vi "Script IO Nodes.vi"(5 "Device Info":T1, 6 "Number of SPI Buses":i32, 7 "Curent Bus Path":path, 8 "error in (no error)":errorcluster, 9 "Device Channels":i32[](array[numeric]), 11 "LabVIEW Project to Script":path) -> (0 "error out":errorcluster, 3 "New Node Paths":path[](array[path]))   [LabVIEW 2014, in "Initialization and IO Node Scripting.lvlib"]
uses:
  Initialization and IO Node Scripting.lvlib
  State Machine/Controls/Bus Information.ctl
  State Machine/Controls/Device Information.ctl
  State Machine/Controls/Pin Information.ctl
  State Machine/Controls/Values for Naming.ctl
panel:
  in  "New Virtual Folder":refnum<vi>
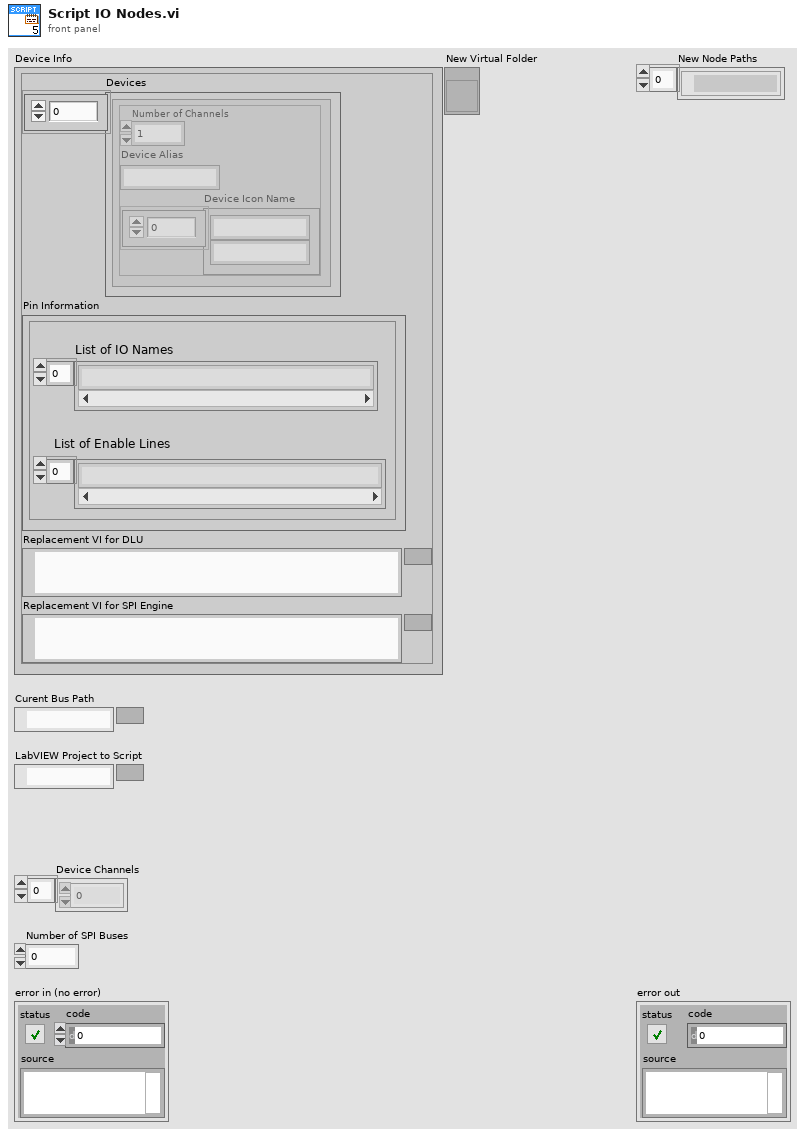
[diagram p1: front panel]
types:
  T1 = typedef "Initialization and IO Node Scripting.lvlib/Bus Information.ctl" = cluster{"Devices":T2[], "Pin Information":T3, "Replacement VI for DLU":path, "Replacement VI for SPI Engine":path}
  T2 = typedef "Device Information.ctl" = cluster{"Number of Channels":i32, "Device Alias":string, "Device Icon Name":string[]}
  T3 = typedef "Pin Information.ctl" = cluster{"List of IO Names":string[], "List of Enable Lines":string[]}
  T4 = typedef "Initialization and IO Node Scripting.lvlib/Values for Naming.ctl" = cluster{"Bus Number":i32, "Device Number":i32, "Channel Number":i32}
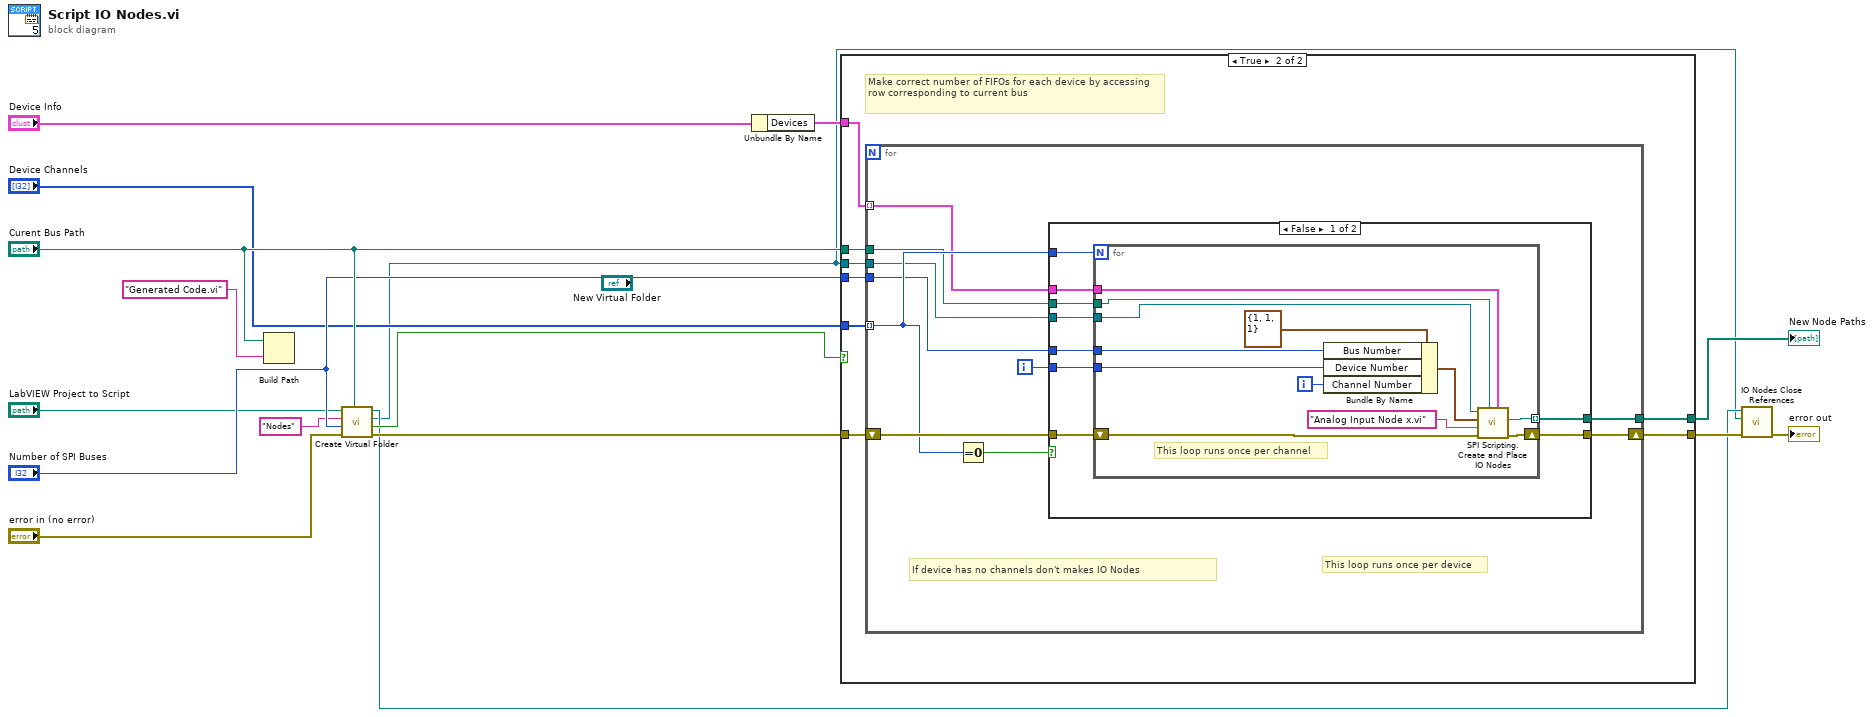
[diagram p0: block diagram]
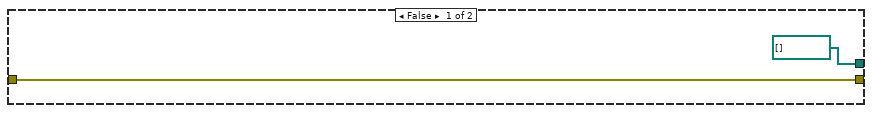
[diagram p2: hidden frame]
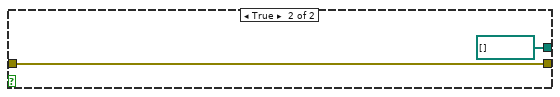
[diagram p3: hidden frame]
diagram:
  n1 = Build Path(base path="Curent Bus Path", name or relative path="Generated Code.vi") -> ()  [unwired: 1 out]
  n2 = call "Create Virtual Folder.vi"("Curent Bus Path"="Curent Bus Path", "error in"="error in (no error)", "Bus Number"="Number of SPI Buses", "Virtual Folder Name"="Nodes", "Path to Project"="LabVIEW Project to Script") -> ("error out"=w3:errorcluster, "FPGA Target Found"=w8:bool, "New Virtual Folder"=w1:refnum<vi>, "Project:Open"=w2:refnum<vi>)  [unwired: 3 in]
  n3 = Unbundle By Name("Device Info") -> ("Devices"=w16:T2[])
  n4 = case shown="True" w8 {
    tunnel: [w17 w26] -> w12
    tunnel: "Device Channels" -> [_ w22]
    tunnel: "Number of SPI Buses" -> [_ w25]
    tunnel: "Curent Bus Path" -> [_ w24]
    tunnel: w1 -> [_ w23]
    tunnel: w16 -> [_ w21]
    tunnel: [path[] [] w20] -> w4
    tunnel: w3 -> [w17 w19]
    frame False {
    }
    frame True {
      # "Make correct number of FIFOs for each device by accessing row corresponding to current bus"
      n5 = for {
        shift-right: [w36] -> w26
        shift-left: w19 -> [w35]
        tunnel: w22 -> [w32] mode=indexing
        tunnel: w25 -> [w31]
        tunnel: w24 -> [w30]
        tunnel: w23 -> [w29]
        tunnel: w21 -> [w28] mode=indexing
        tunnel: [w27] -> w20
        i -> [w33]
        # "This loop runs once per device"
        # "If device has no channels don't makes IO Nodes"
        n6 = Equal To 0?(x=w32) -> (x = 0?=w34:bool)
        n7 = case shown="False" w34 {
          tunnel: [w45 w59] -> w36
          tunnel: w35 -> [w44 w59]
          tunnel: w33 -> [w43 _]
          tunnel: w32 -> [w42 _]
          tunnel: w31 -> [w41 _]
          tunnel: w30 -> [w40 _]
          tunnel: w29 -> [w39 _]
          tunnel: w28 -> [w38 _]
          tunnel: [w37 path[] []] -> w27
          frame False {
            n8 = for {
              N: w42 -> [_]
              shift-right: [w56] -> w45
              shift-left: w44 -> [w57]
              tunnel: w43 -> [w53]
              tunnel: w41 -> [w54]
              tunnel: w40 -> [w55]
              tunnel: w39 -> [w50]
              tunnel: w38 -> [w47]
              tunnel: [w46] -> w37 mode=indexing
              i -> [w52]
              # "This loop runs once per channel"
              n9 = Bundle By Name(cluster=T4 {"Bus Number"=1, "Device Number"=1, "Channel Number"=1} ("Values for Naming"), "Bus Number"=w54, "Device Number"=w53, "Channel Number"=w52) -> (w49:T4)
              n10 = call "SPI Scripting.Create and Place IO Nodes.vi"("Device Information"=w47, "Current Bus Path"=w55, "error in"=w57, "Path to Analog Node Template"="Analog Input Node x.vi", "Values for Naming"=w49, "Virtual Folder"=w50) -> ("error out"=w56:errorcluster, "Path to New Node"=w46:path)  [unwired: 3 in, 1 out]
            }
          }
          frame True {
          }
        }
      }
    }
  }
  "New Node Paths" <- w4
  n11 = call "IO Nodes Close References.vi"("error in (no error)"=w12, "Virtual Folder"=w1, "Project in"=w2) -> ("error out"=→"error out":errorcluster)  [unwired: 8 in]
